vi "p2.vi"() -> ()   [LabVIEW 2021, in "d10.lvlib"]
uses:
  d10.lvlib
  AOC/AOC.lvlib
panel:
  out "XY Graph":cluster{i64, i64}[](graph)=[{1, 0}, {2, 0}, {3, 0}, {8, 0}, {12, 0}, {16, 0}, {18, 0}, {20, 0}, {21, 0}, {26, 0}, {30, 0}, {35, 0}, {0, -1}, {8, -1}, {10, -1}, {13, -1}, {15, -1}, {20, -1}, {28, -1}, {30, -1}, {35, -1}, {38, -1}, {0, -2}, {2, -2}, {8, -2}, {10, -2}, {15, -2}, {16, -2}, {17, -2}, {23, -2}, {25, -2}, {35, -2}, {37, -2}, {8, -3}, {10, -3}, {15, -3}, {20, -3}, {22, -3}, {28, -3}, {30, -3}, {35, -3}, {5, -4}, {13, -4}, {15, -4}, {25, -4}, {35, -4}, {0, -5}, {2, -5}, {6, -5}, {7, -5}, {11, -5}, {15, -5}, {27, -5}, {31, -5}, {33, -5}, {35, -5}, {38, -5}, {0, 0}, {7, 0}, {11, 0}, {15, 0}, {17, 0}, {22, 0}, {27, 0}, {38, 0}, {23, -1}, {25, -1}, {1, -2}, {20, -2}, {30, -2}, {36, -2}, {38, -2}, {0, -3}, {21, -3}, {25, -3}, {27, -3}, {38, -3}, {0, -4}, {8, -4}, {10, -4}, {20, -4}, {28, -4}, {30, -4}, {38, -4}, {1, -5}, {3, -5}, {12, -5}, {20, -5}, {26, -5}, {28, -5}, {30, -5}, {32, -5}]
  in  "Example":string="addx 15\naddx -11\naddx 6\naddx -3\naddx 5\naddx -1\naddx -8\naddx 13\naddx 4\nnoop\naddx -1\naddx 5\naddx -1\naddx 5\naddx -1\naddx 5\naddx -1\naddx 5\naddx -1\naddx -35\naddx 1\naddx 24\naddx -19\naddx 1\naddx 16\naddx -11\nnoop\nnoop\naddx 21\naddx -15\nnoop\nnoop\naddx -3\naddx 9\naddx 1\naddx -3\naddx 8\naddx 1\naddx 5\nnoop\nnoop\nnoop\nnoop\nnoop\naddx -36\nnoop\naddx 1\naddx 7\nnoop\nnoop\nnoop\naddx 2\naddx 6\nnoop\nnoop\nnoop\nnoop\nnoop\naddx 1\nnoop\nnoop\naddx 7\naddx 1\nnoop\naddx -13\naddx 13\naddx 7\nnoop\naddx 1\naddx -33\nnoop\nnoop\nnoop\naddx 2\nnoop\nnoop\nnoop\naddx 8\nnoop\naddx -1\naddx 2\naddx 1\nnoop\naddx 17\naddx -9\naddx 1\naddx 1\naddx -3\naddx 11\nnoop\nnoop\naddx 1\nnoop\naddx 1\nnoop\nnoop\naddx -13\naddx -19\naddx 1\naddx 3\naddx 26\naddx -30\naddx 12\naddx -1\naddx 3\naddx 1\nnoop\nnoop\nnoop\naddx -9\naddx 18\naddx 1\naddx 2\nnoop\nnoop\naddx 9\nnoop\nnoop\nnoop\naddx -1\naddx 2\naddx -37\naddx 1\naddx 3\nnoop\naddx 15\naddx -21\naddx 22\naddx -6\naddx 1\nnoop\naddx 2\naddx 1\nnoop\naddx -10\nnoop\nnoop\naddx 20\naddx 1\naddx 2\naddx 2\naddx -6\naddx -11\nnoop\nnoop\nnoop"
  in  "Example":bool
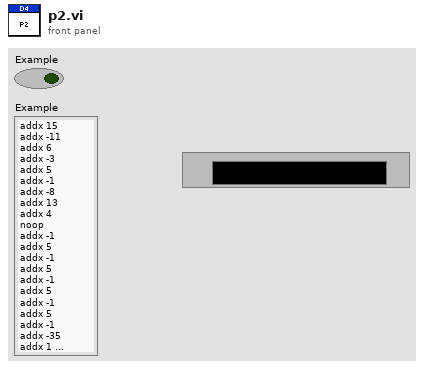
[diagram p1: front panel]
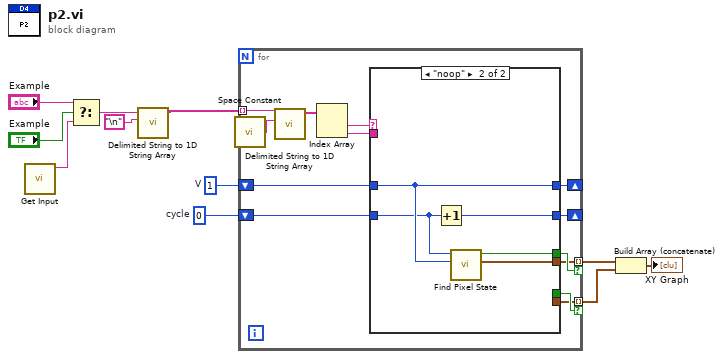
[diagram p0: block diagram]
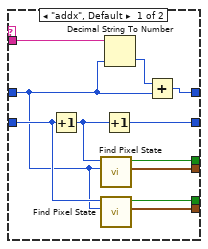
[diagram p2: hidden frame]
diagram:
  w5 = i64 0  # cycle
  w6 = i64 1  # V
  n1 = call "Get Input.vi"() -> ("Input"=w11:string)  [unwired: 11 in]
  n2 = Select(t="Example", s="Example", f=w11) -> (s? t:f=w10:string)
  n3 = call <vilib>:"Delimited String to 1D String Array.vi"("delimiter"="\n", "delimited string"=w10) -> ("string array"=w4:string[])  [unwired: 9 in]
  n4 = for {
    tunnel: w4 -> [w24] mode=indexing
    shift-right: [w18] -> _
    shift-left: w6 -> [w20]
    shift-right: [w17] -> _
    shift-left: w5 -> [w19]
    tunnel: [w13] -> w3 mode=indexing if=w15
    tunnel: [w12] -> w2 mode=indexing if=w14
    n5 = call <vilib>:"Space Constant.vi"() -> ("String"=w23:string)
    n6 = call <vilib>:"Delimited String to 1D String Array.vi"("delimiter"=w23, "delimited string"=w24) -> ("string array"=w22:string[])  [unwired: 9 in]
    n7 = Index Array(array=w22) -> (element #1=w21:string, element #2=w16:string)  [unwired: 2 in]
    n8 = case shown="\"noop\"" w21 {
      tunnel: w20 -> [w27 w39]
      tunnel: w19 -> [w28 w38]
      tunnel: [w31 w39] -> w18
      tunnel: [w33 w40] -> w17
      tunnel: w16 -> [w35 _]
      tunnel: [w32 w36] -> w15
      tunnel: [w25 _] -> w14
      tunnel: [w29 w37] -> w13
      tunnel: [w26 _] -> w12
      frame "addx", Default {
        n9 = Increment(x=w28) -> (x+1=w30:i64)
        n10 = call "Find Pixel State.vi"("V"=w27, "cycle"=w30) -> ("Position"=w29:cluster{i64, i64}, "State"=w32:bool)  [unwired: 8 in]
        n11 = call "Find Pixel State.vi"("V"=w27, "cycle"=w28) -> ("Position"=w26:cluster{i64, i64}, "State"=w25:bool)  [unwired: 8 in]
        n12 = Increment(x=w30) -> (x+1=w33:i64)
        n13 = Decimal String To Number(string=w35, default (0L)=w27) -> (number=w34:i64)  [unwired: 1 in, 1 out]
        n14 = Add(x=w34, y=w27) -> (x+y=w31:i64)
      }
      frame "noop" {
        n15 = Increment(x=w38) -> (x+1=w40:i64)
        n16 = call "Find Pixel State.vi"("V"=w39, "cycle"=w38) -> ("Position"=w37:cluster{i64, i64}, "State"=w36:bool)  [unwired: 8 in]
      }
    }
  }
  n17 = Build Array (concatenate)(w3, w2) -> (→"XY Graph":cluster{i64, i64}[])
